vi "GEvt-Generate Module Created Log.vi"(0 "CSM Global Log Event":T4, 6 "Name (\"\" to Use UUID)":string, 7 "Created?":bool, 10 "CSM:LogFilter.lvclass":refnum<class "LogFilter.lvclass">) -> (14 "CSM Global Log Event Out":T4, 16 "Event Data":T1={"Name (\"\" to Use UUID)"="", "Current State"="", "Arguments"="", "Source Message"={"‘State"="", "’Arguments"="", "’Error"={"status"=FALSE, "code"=0, "source"=""}}, "Source Module"="", "Complete(T)/Start(F)"=FALSE, "LogType"=enum."State Change", "Time Stamp"=timestamp(0 s since 1904-01-01)})   [LabVIEW 2017, in "Communicable State Machine.lvlib"]
doc: "### GEvt-Generate Module Created Log.vi\n\n-- <b>Controls</b> --\n- <b>CSM Global Log Event</b>:\n- <b>Name(\"\" to use uuid)</b>:\n- <b>Created?</b>:\n- <b>CSM:LogFilter.lvclass</b>:\n\n-- <b>Indicators</b> --\n- <b>CSM Global Log Event out</b>:\n- <b>event data</b>:"
uses:
  Communicable State Machine.lvlib
  GEvt-Refs.ctl
  Typedef/_CSM_GlobalLog_MSG.ctl
  Typedef/_CSM_Response Source Message.ctl
  Typedef/_CSM_GlobalLog_MSG_TYPE.ctl
  LogFilter/LogFilter.lvclass
  LogFilter/LogFilter - Check.vi
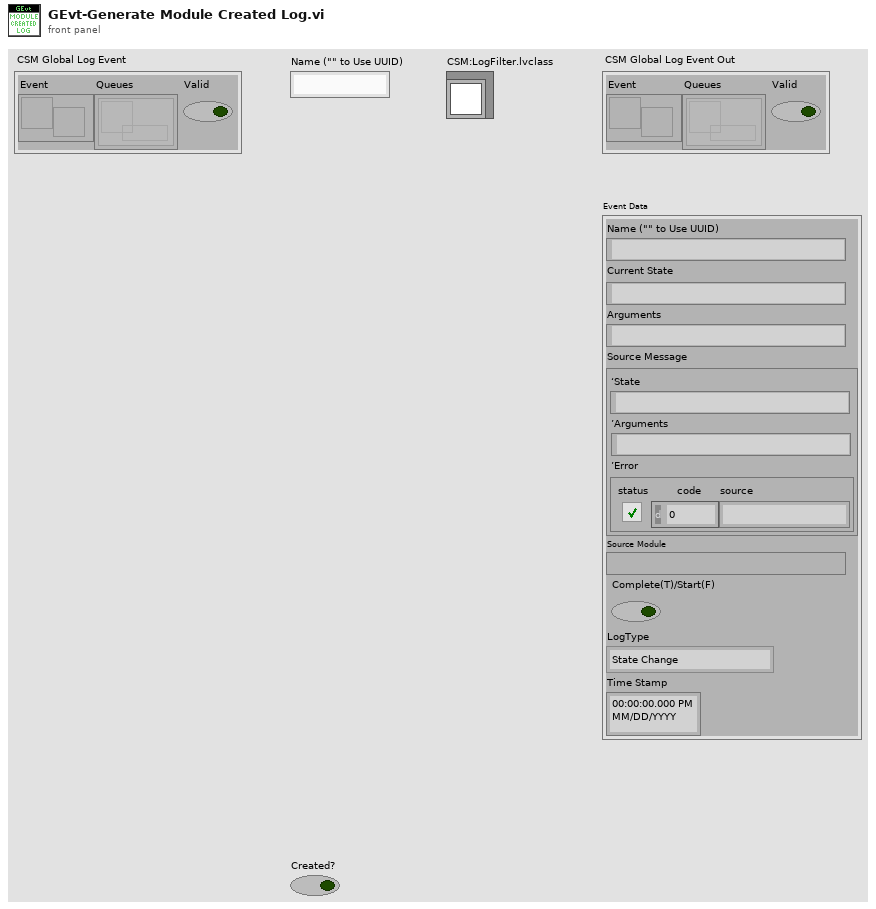
[diagram p1: front panel]
types:
  T1 = typedef "Communicable State Machine.lvlib/_CSM_GlobalLog_MSG.ctl" = cluster{"Name (\"\" to Use UUID)":string, "Current State":string, "Arguments":string, "Source Message":T2, "Source Module":string, "Complete(T)/Start(F)":bool, "LogType":T3, "Time Stamp":timestamp}
  T2 = typedef "Communicable State Machine.lvlib/_CSM_Response Source Message.ctl" = cluster{"‘State":string, "’Arguments":string, "’Error":errorcluster}
  T3 = typedef "Communicable State Machine.lvlib/_CSM_GlobalLog_MSG_TYPE.ctl" = enum16{"User Log", "State Change", "Status", "Interrupt", "Register", "Unregister", "Error Log", "Module Created", "Module Destroyed"}
  T4 = typedef "Communicable State Machine.lvlib/GEvt-Refs.ctl" = cluster{"Event":refnum<user-event>, "Queues":refnum<queue>[], "Valid":bool}
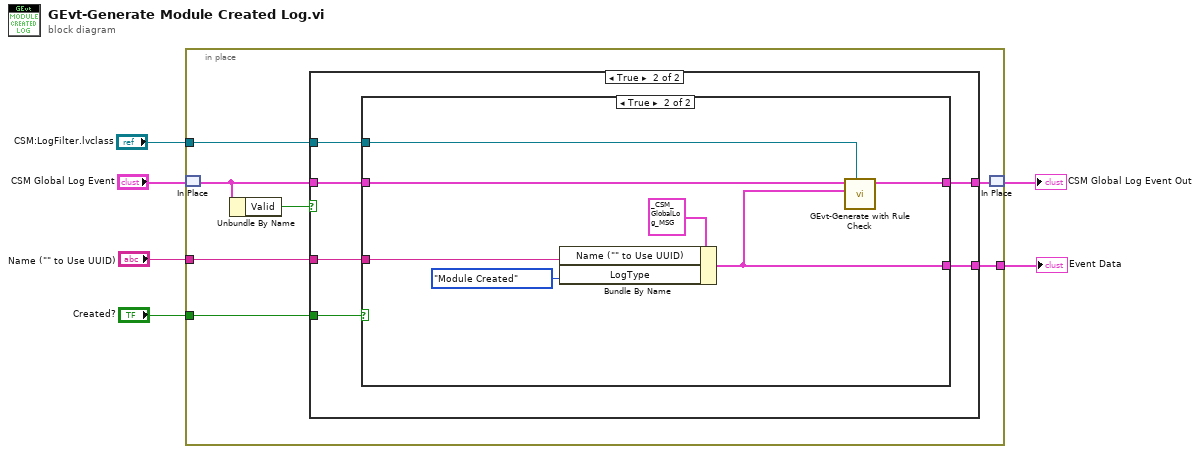
[diagram p0: block diagram]
diagram:
  n1 = in-place {
    in-place-border: [w12] -> w4
    in-place-border: "Created?" -> [w11]
    in-place-border: "Name (\"\" to Use UUID)" -> [w10]
    in-place-border: "CSM:LogFilter.lvclass" -> [w9]
    n2 = in-place-match #1("CSM Global Log Event") -> (w8:T4)
    n3 = Unbundle By Name(w8) -> ("Valid"=w7:bool)
    n4 = case shown="True" w7 {
      tunnel: w8 -> [w14 w20]
      tunnel: [w14 w19] -> w13
      tunnel: [_ w18] -> w12
      tunnel: w11 -> [_ w17]
      tunnel: w10 -> [_ w16]
      tunnel: w9 -> [_ w15]
      frame False {
      }
      frame True {
        n5 = case shown="True" w17 {
          tunnel: w20 -> [w21 w28]
          tunnel: [w21 w27] -> w19
          tunnel: [_ w23] -> w18
          tunnel: w16 -> [_ w24]
          tunnel: w15 -> [_ w22]
          frame False {
          }
          frame True {
            n6 = Bundle By Name(cluster=T1 {"Name (\"\" to Use UUID)"="", "Current State"="", "Arguments"="", "Source Message"={"‘State"="", "’Arguments"="", "’Error"={"status"=FALSE, "code"=0, "source"=""}}, "Source Module"="", "Complete(T)/Start(F)"=FALSE, "LogType"=enum."State Change", "Time Stamp"=timestamp(0 s since 1904-01-01)} ("event data"), "Name (\"\" to Use UUID)"=w24, "LogType"=_CSM_GlobalLog_MSG_TYPE."Module Created" ("Type")) -> (w23:T1)
            n7 = call "GEvt-Generate with Rule Check.vi"("LogFilter In"=w22, "Event Data"=w23, "CSM Global Log Event In"=w28) -> ("CSM Global Log Event Out"=w27:T4)  [unwired: 8 in]
          }
        }
      }
    }
    n8 = in-place-match #1(w13) -> (→"CSM Global Log Event Out":T4)
  }
  "Event Data" <- w4
